vi "Destroy.vi"(8 "error in (no error)":errorcluster, 11 "Status Updater in":refnum<class "Status Events.lvclass">) -> (0 "error out":errorcluster)   [LabVIEW 2014]
uses:
  Status Events.lvclass
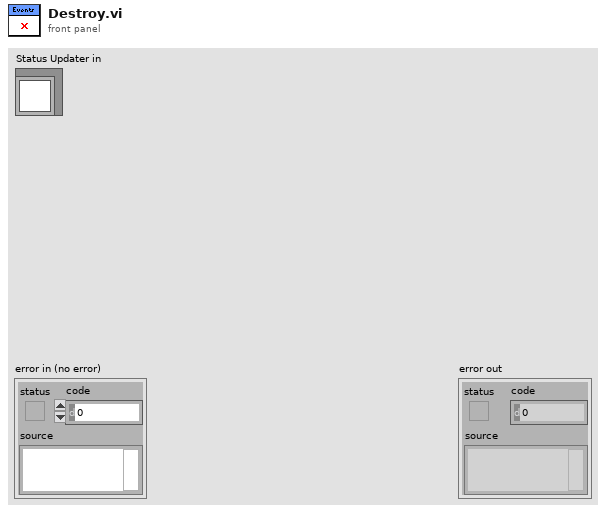
[diagram p1: front panel]
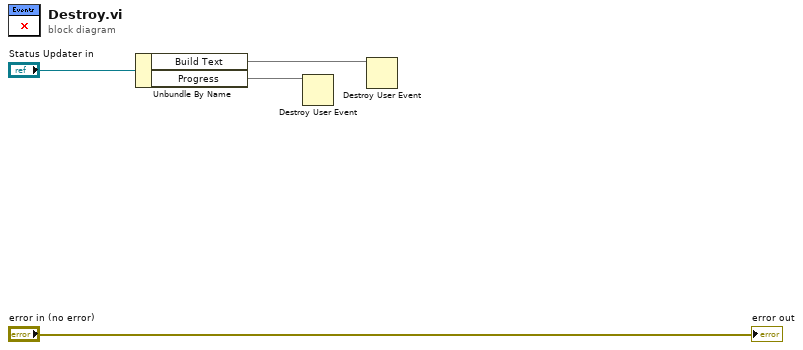
[diagram p0: block diagram]
diagram:
  n1 = Unbundle By Name("Status Updater in") -> ("Build Text"=w3, "Progress"=w2)
  n2 = Destroy User Event(user event=w2) -> ()  [unwired: 1 in, 1 out]
  n3 = Destroy User Event(user event=w3) -> ()  [unwired: 1 in, 1 out]
  "error out" <- "error in (no error)"
